vi "Parse ACL Device Reading.vi"(8 "error in (no error)":errorcluster, 11 "Reading String":string="<?xml version=\"1.0\" encoding=\"ISO-8859-1\" standalone=\"no\" ?>\n<methodResponse>\n\n  <params>\n    <param>\n      <value>\n        <struct>\n          <member>\n            <name>status</name>\n            <value>\n              <int>0</int>\n            </value>\n          </member>\n          <member>\n            <name>scaled</name>\n            <value>\n              <double>0.9992975666172701</double>\n            </value>\n          </member>\n          <member>\n            <name>units</name>\n            <value>Torr</value>\n          </member>\n          <member>\n            <name>name</name>\n            <value>e:201vac</value>\n          </member>\n        </struct>\n      </value>\n    </param>\n  </params>\n\n</methodResponse>\n") -> (0 "error out":errorcluster, 3 "Reading":T1)   [LabVIEW 2013, in "Controls Log Monitor.lvlib"]
uses:
  MTA Shift Toolbox/Controls Log Monitor.lvlib
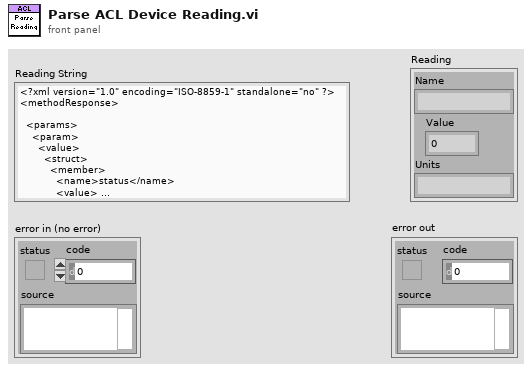
[diagram p1: front panel]
types:
  T1 = cluster{"Name":string, "Value":dbl, "Units":string}
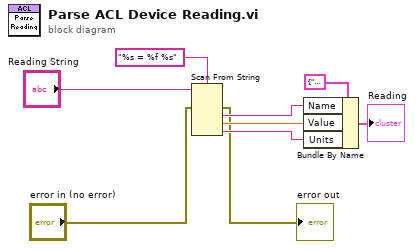
[diagram p0: block diagram]
diagram:
  n1 = Scan From String(format string="%s = %f %s", input string="Reading String", error in="error in (no error)") -> (error out=→"error out":errorcluster, output 1=w5:string, output 2=w6:dbl, output 3=w4:string)  [unwired: 4 in, 2 out]
  n2 = Bundle By Name(cluster=T1 {"Name"="", "Value"=0.0, "Units"=""} ("Reading"), "Name"=w5, "Value"=w6, "Units"=w4) -> (→"Reading":T1)
